vi "Single SSC DCPower Get Aperture Times in Seconds.vi"(0 "DCPower SSC in":T1, 11 "error in":errorcluster) -> (4 "DCPower SSC out":T1, 6 "Actual Aperture Times (s)":dbl format="%#_6p", 15 "error out":errorcluster)   [LabVIEW 2020]
doc: "This VI gets the measurement aperture time of the session in seconds (if it was set in units of PLCs, it converts it to seconds)."
uses:
  SSC DCPower.ctl
  <instrlib>/niDCPower/nidcpower.llb/niDCPower Aperture Time Units.ctl
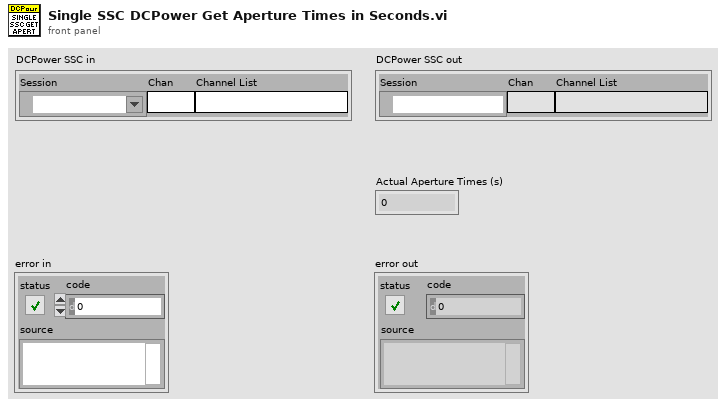
[diagram p1: front panel]
types:
  T1 = typedef "SSC DCPower.ctl" = cluster{"Session":refnum<k15>, "Chan":string, "Channel List":string}
  T2 = typedef "niDCPower Aperture Time Units.ctl" = i32
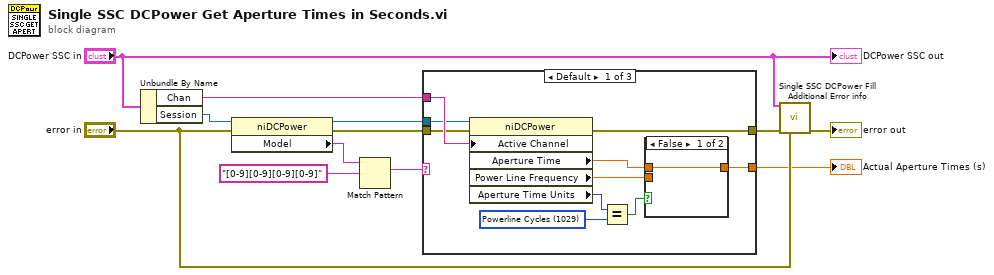
[diagram p0: block diagram]
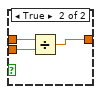
[diagram p2: hidden frame]
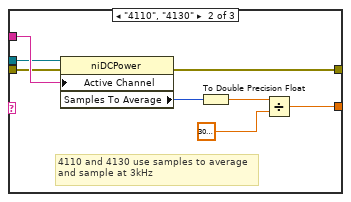
[diagram p3: hidden frame]
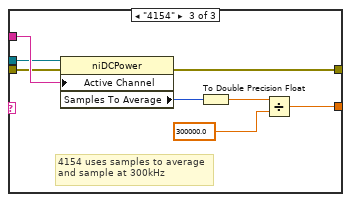
[diagram p4: hidden frame]
diagram:
  n1 = Unbundle By Name("DCPower SSC in") -> ("Chan"=w7:string, "Session"=w4:refnum<k15>)
  n2 = property class="niDCPower"(reference=w4, error in="error in") -> (reference out=w5:refnum<k15>, error out=w6:errorcluster, "Model"=w2:string)
  n3 = Match Pattern(string=w2, regular expression="[0-9][0-9][0-9][0-9]") -> (match substring=w1:string)  [unwired: 1 in, 3 out]
  n4 = case shown="Default" w1 {
    tunnel: [w22 w34 w42] -> w8
    tunnel: [w18 w29 w37] -> w10
    tunnel: w7 -> [w16 w33 w41]
    tunnel: w6 -> [w14 w32 w40]
    tunnel: w5 -> [w13 w31 w39]
    frame Default {
      w21 = T2 1029 items=["Seconds"=1028, "Powerline Cycles"=1029] ("aperture time units")
      n5 = property class="niDCPower"(reference=w13, error in=w14, "Active Channel"=w16) -> (error out=w22:errorcluster, "Aperture Time"=w19:dbl, "Power Line Frequency"=w17:dbl, "Aperture Time Units"=w20:i32)  [unwired: 1 out]
      n6 = Equal?(x=w20, y=w21) -> (x = y?=w15:bool)
      n7 = case shown="False" w15 {
        tunnel: w19 -> [w23 w25]
        tunnel: [w23 w26] -> w18
        tunnel: w17 -> [_ w24]
        frame False {
        }
        frame True {
          n8 = Divide(x=w25, y=w24) -> (x/y=w26:dbl)
        }
      }
    }
    frame "4110", "4130" {
      # "4110 and 4130 use samples to average\nand sample at 3kHz"
      n9 = property class="niDCPower"(reference=w31, error in=w32, "Active Channel"=w33) -> (error out=w34:errorcluster, "Samples To Average"=w30:i32)  [unwired: 1 out]
      n10 = To Double Precision Float(number=w30) -> (double precision float=w27:dbl)
      n11 = Divide(x=w27, y=3000.0) -> (x/y=w29:dbl)
    }
    frame "4154" {
      # "4154 uses samples to average\nand sample at 300kHz"
      n12 = property class="niDCPower"(reference=w39, error in=w40, "Active Channel"=w41) -> (error out=w42:errorcluster, "Samples To Average"=w38:i32)  [unwired: 1 out]
      n13 = To Double Precision Float(number=w38) -> (double precision float=w35:dbl)
      n14 = Divide(x=w35, y=300000.0) -> (x/y=w37:dbl)
    }
  }
  "Actual Aperture Times (s)" <- w10
  n15 = call "Single SSC DCPower Fill Additional Error info.vi"("DCPower SSC in"="DCPower SSC in", "error in"=w8, "previous error in"="error in") -> ("error out"=→"error out":errorcluster)  [unwired: 12 in]
  "DCPower SSC out" <- "DCPower SSC in"
